vi "InternDay3_Template.vi"() -> ()   [LabVIEW 2026]
uses:
  <vilib>/numeric/Random Number (Range) U64.vi
panel:
  in  "Stop":bool
  in  "Buttons":bool[](array[boolean])
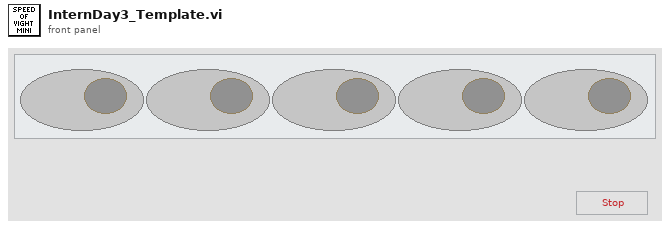
[diagram p1: front panel]
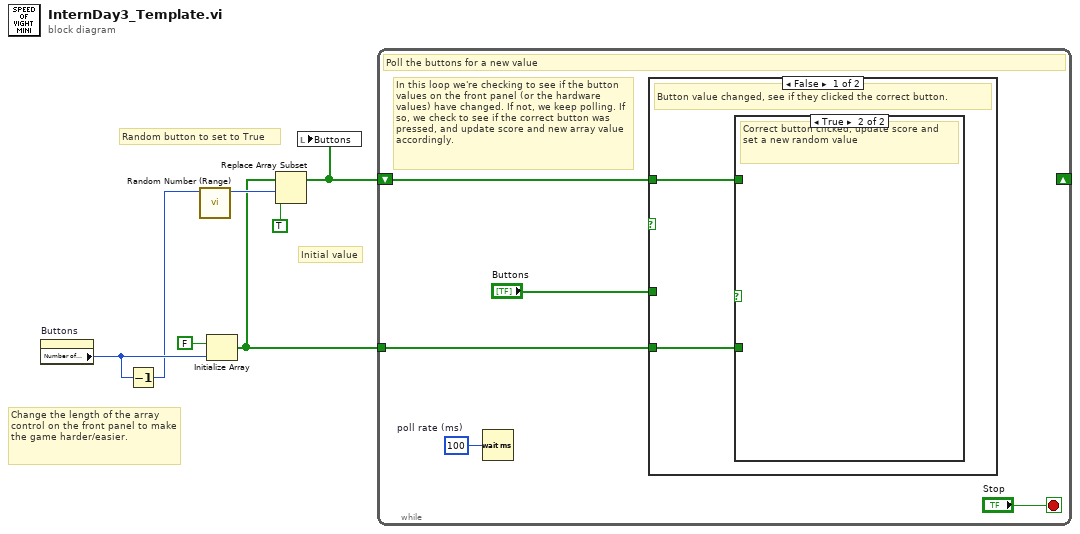
[diagram p0: block diagram]
diagram:
  # "Random button to set to True"
  # "Initial value"
  # "Change the length of the array control on the front panel to make the game harder/easier."
  n1 = property on="Buttons" class="Arr (strict)"() -> ("Number of Columns"=w2:u32)  [unwired: 2 in, 2 out]
  n2 = Decrement(x=w2) -> (x-1=w1:u32)
  n3 = call-poly <vilib>:"Random Number (Range).vi"("upper bound (100)"=w1) -> ("number"=w6:u64)  [unwired: 10 in]
  n4 = Initialize Array(FALSE, w2) -> (w5:bool[])
  n5 = Replace Array Subset(array=w5, new element=TRUE ("new element/subarray"), index=w6) -> (w3:bool[])
  n6 = local write "Buttons"(w3) -> ()
  n7 = while {
    tunnel: w5 -> [w9]
    shift-right: _ -> [_]
    shift-left: w3 -> [w10]
    stop <- "Stop" stop-if-true
    w11 = u32 100  # poll rate (ms)
    # "In this loop we're checking to see if the button values on the front panel (or the hardware values) have changed. If not, we keep polling. If so, we check to see if the correct button was pressed, and update score and new array value accordingly."
    # "Poll the buttons for a new value"
    n8 = Wait (ms)(milliseconds to wait=w11) -> ()  [unwired: 1 out]
    n9 = case shown="False" {
      selector: _ -> [_ _]
      tunnel: w10 -> [w13 _]
      tunnel: w9 -> [w14 _]
      tunnel: "Buttons" -> [_ _]
      frame False {
        # "Button value changed, see if they clicked the correct button."
        n10 = case shown="True" {
          selector: _ -> [_ _]
          tunnel: w14 -> [_ _]
          tunnel: w13 -> [_ _]
          frame False {
            # "Wrong button clicked. Do nothing for now....."
          }
          frame True {
            # "Correct button clicked, update score and set a new random value"
          }
        }
      }
      frame True {
        # "Button value did not change"
      }
    }
  }
